vi "Insight_Initiate_Fixed_Wavelength.vi"(8 "error in (no error)":errorcluster, 9 "Mode (Read / Write)":enum8{"Write", "Read"}(ring), 11 "telnet connection":T1) -> (0 "error out":errorcluster, 1 "response data":string, 2 "Fixed Wavelength Mode?":enum16{"Off", "On"}(ring), 3 "telnet  connection out":T1)   [LabVIEW 2011]
doc: "Insight Photonic Solutions\n\nThis VI initiates the Fixed Wavelength Mode of the laser, or allows the user to query the state. The output of the laser is turned on and the laser is set to a fixed wavelength value.\n\nInputs:\nRead/Write : command or query the state of Fixed Wavelength Mode\n\nOutputs:\nFixed Wavelength Mode? - On or Off\n\nver 1.0 - original release"
uses:
  Telnet Session.ctl
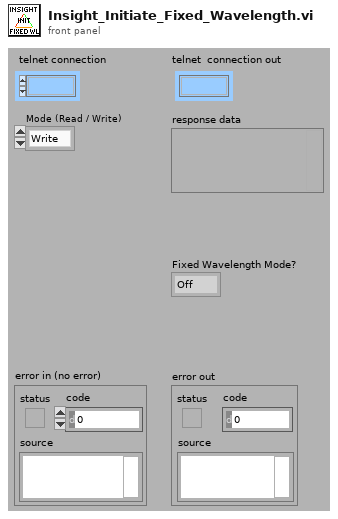
[diagram p1: front panel]
types:
  T1 = typedef "Telnet Session.ctl" = refnum<k1>
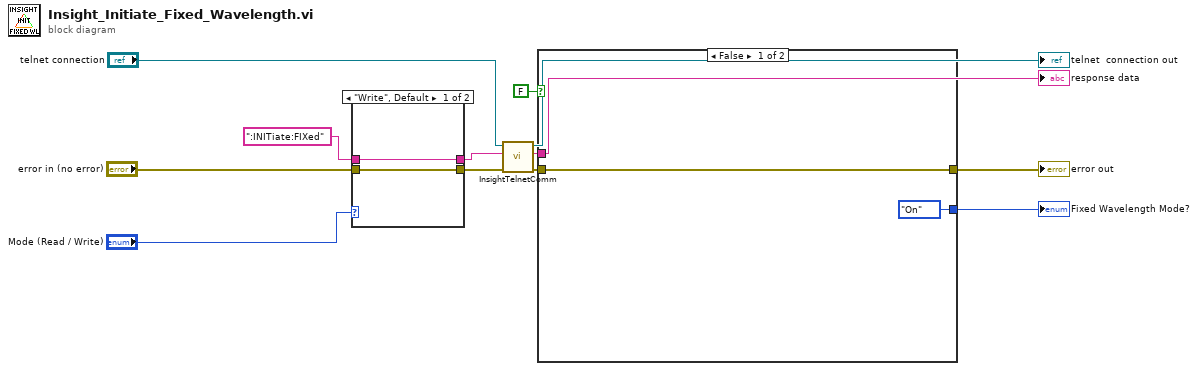
[diagram p0: block diagram]
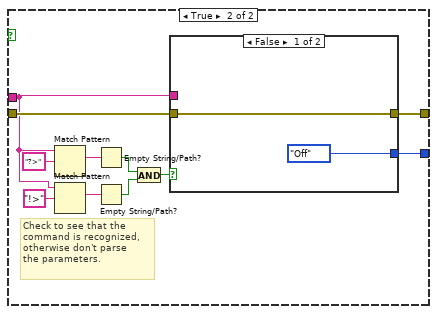
[diagram p2: hidden frame]
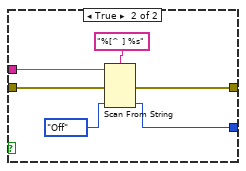
[diagram p3: hidden frame]
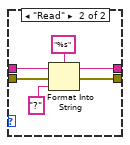
[diagram p4: hidden frame]
diagram:
  n1 = case shown="\"Write\", Default" "Mode (Read / Write)" {
    tunnel: [w13 w16] -> w6
    tunnel: "error in (no error)" -> [w13 w15]
    tunnel: ":INITiate:FIXed" ("String") -> [w14 w18]
    tunnel: [w14 w17] -> w9
    frame "Write", Default {
    }
    frame "Read" {
      n2 = Format Into String(format string="%s", initial string=w18, error in=w15, "?" ("input 1")) -> (resulting string=w17:string, error out=w16:errorcluster)
    }
  }
  n3 = call "InsightTelnetComm.vi"("error in"=w6, "write buffer (\"\")"=w9, "telnet connection"="telnet connection") -> ("error out"=w4:errorcluster, "response data"=w3:string, "telnet  connection out"=→"telnet  connection out":T1)  [unwired: 4 in]
  "response data" <- w3
  n4 = case shown="False" FALSE {
    tunnel: [w22 w33] -> w5
    tunnel: w4 -> [w22 w32]
    tunnel: w3 -> [_ w24]
    tunnel: [enum16{"Off", "On"}."On" ("Fixed Wavelength Mode?") w23] -> w2
    frame False {
    }
    frame True {
      # "Check to see that the \ncommand is recognized,\notherwise don't parse \nthe parameters."
      n5 = Match Pattern(string=w24, regular expression="?>") -> (match substring=w30:string)  [unwired: 1 in, 3 out]
      n6 = Match Pattern(string=w24, regular expression="!>") -> (match substring=w29:string)  [unwired: 1 in, 3 out]
      n7 = Empty String/Path?(string/path=w30) -> (empty?=w27:bool)
      n8 = Empty String/Path?(string/path=w29) -> (empty?=w26:bool)
      n9 = And(x=w27, y=w26) -> (x .and. y?=w25:bool)
      n10 = case shown="False" w25 {
        tunnel: [w35 w38] -> w33
        tunnel: w32 -> [w35 w39]
        tunnel: w24 -> [_ w40]
        tunnel: [enum16{"Off", "On"}."Off" ("Fixed Wavelength Mode?") w37] -> w23
        frame False {
        }
        frame True {
          n11 = Scan From String(format string="%[^ ] %s", input string=w40, error in=w39, default 2=enum16{"Off", "On"}."Off" ("Fixed Wavelength Mode?")) -> (error out=w38:errorcluster, output 2=w37:enum16{"Off", "On"})  [unwired: 3 in, 2 out]
        }
      }
    }
  }
  "error out" <- w5
  "Fixed Wavelength Mode?" <- w2
